vi "VI Tree.vi"   [LabVIEW 2021, in "UserEvent.lvlib"]
uses:
  UserEvent.lvlib
  4a2ca208-d08a-422b-8799-d4cf94fa1625.vi
  ae7c6603-eda3-48db-b0d2-d576bcba6bd2.vi
  7e40b7d5-d22b-4c9e-9579-184d2a0dae0b.vi
  726e3b52-0671-4950-8a71-d94978cc7dba.vi
  4a11929e-71d2-4f44-a657-a59de206d2c9.vi
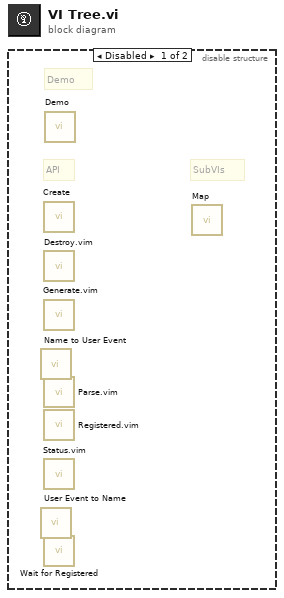
[diagram p0: block diagram]
diagram:
  n1 = disable-structure shown="Disabled" {
    frame Disabled {
      # "SubVIs"
      # "API"
      # "Demo"
      n2 = call "Name to User Event.vi"() -> ()  [unwired: 7 in, 3 out]
      n3 = call "User Event to Name.vi"() -> ()  [unwired: 7 in, 3 out]
      n4 = call "Create.vi"() -> ()  [unwired: 8 in, 4 out]
      n5 = call "Destroy.vim"() -> ()  [unwired: 10 in, 2 out]
      n6 = call "Generate.vim"() -> ()  [unwired: 10 in, 2 out]
      n7 = call "Parse.vim"() -> ()  [unwired: 10 in, 2 out]
      n8 = call "Registered.vim"() -> ()  [unwired: 10 in, 2 out]
      n9 = call "Status.vim"() -> ()  [unwired: 7 in, 5 out]
      n10 = call "Wait for Registered.vi"() -> ()  [unwired: 9 in, 3 out]
      n11 = call "Demo.vi"() -> ()  [unwired: 12 in]
      n12 = call "Map.vi"() -> ()  [unwired: 8 in, 4 out]
    }
    frame Enabled {
    }
  }
